vi "SL TAGS Return Unit of Measure Abbreviation.vi"(4 "Unit of Measure":T1=enum."Hour") -> (1 "Seeq Unit of Measure Abbreviation":string)   [LabVIEW 2017, in "EEISysLink.lvclass"]
doc: "Convert selected units to Seeq supported unit abbreviation string\n\nJames Tillett\nEndeavor Engineering Inc.\nwww.endeavoreng.com"
uses:
  EEISysLink.lvclass
  Controls/SL Tag Unit of Measure.ctl
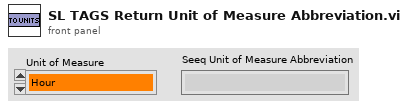
[diagram p1: front panel]
types:
  T1 = typedef "EEISysLink.lvclass/SL Tag Unit of Measure.ctl" = enum16{"no units", "Second", "Hour", "Minute", "Day", "Year", "Month", "Week", "Foot", "Yard", "Meter", "Centimeter", "Inch", "Mile", "Nautical Mile", "Miles per Hour", "Meters per second", "Square meter", "Cubic meter", "Cubic centimeter", "Cubic inch", "Liter", "Gallon", "Gallons dry US", "Gallon UK", "Percent", "Revolutions per minute", "Revolution", "Degree angle", "Astronomical Unit", "Atom", "Atomic mass", "Bar", "Byte", "C (speed of light)", "Curie", "Decibel", "Electron Volt", "Ounce", "Knot", "G", "Grade", "Are", "Hectare", "Faraday", "Franklin", "Gilbert", "Erg", "Lambert", "Maxwell", "Gauss", "Electron mass", "Kilogram force", "Pound force", "Rad", "Centiradian", "Sphere", "Mach", "Fluid Ounces", "Fluid Ounces UK", "Fahrenheit", "Celsius", "Kelvin", "Rankine", "Gram", "Kilogram", "Pound", "Short/US Ton", "Long/UK ton", "Metric ton", "Mole", "Pounds per square inch", "Inches water column", "Torr", "Millitorr", "Millimeter mercury", "Inches mercury", "Bar (2)", "Atmosphere", "Pascal", "Watt", "kiloWatt", "Horsepower", "Kilowatt Hour", "British thermal units", "Millions of BTU", "Ampere", "Candela", "Radian", "Steradian", "Bit", "Hertz", "Newton", "Joule", "Coulomb", "Volt", "Farad", "Ohm", "Siemens", "Weber", "Tesla", "Henry", "Lumen", "Lux", "Becqueral", "Gray", "Sievert", "Katal", "Angstrom", "Light Year", "Parsec", "Point", "Pixel", "Dyne", "Kilogram force (2)", "Pound force (2)", "Rem", "Rutherford", "Roentgen"}
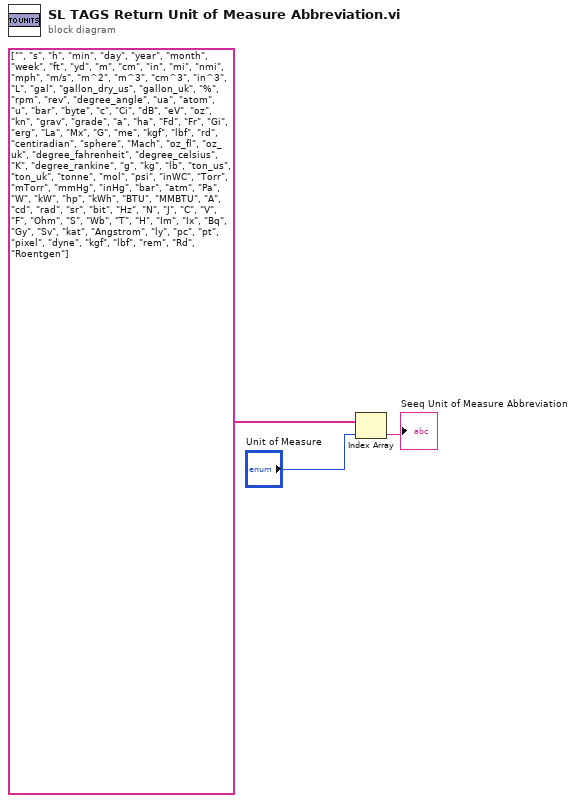
[diagram p0: block diagram]
diagram:
  n1 = Index Array(array=string[] ["", "s", "h", "min", "day", "year", "month", "week", "ft", "yd", "m", "cm", "in", "mi", "nmi", "mph", "m/s", "m^2", "m^3", "cm^3", "in^3", "L", "gal", "gallon_dry_us", "gallon_uk", "%", "rpm", "rev", "degree_angle", "ua", "atom", "u", "bar", "byte", "c", "Ci", "dB", "eV", "oz", "kn", "grav", "grade", "a", "ha", "Fd", "Fr", "Gi", "erg", "La", "Mx", "G", "me", "kgf", "lbf", "rd", "centiradian", "sphere", "Mach", "oz_fl", "oz_uk", "degree_fahrenheit", "degree_celsius", "K", "degree_rankine", "g", "kg", "lb", "ton_us", "ton_uk", "tonne", "mol", "psi", "inWC", "Torr", "mTorr", "mmHg", "inHg", "bar", "atm", "Pa", "W", "kW", "hp", "kWh", "BTU", "MMBTU", "A", "cd", "rad", "sr", "bit", "Hz", "N", "J", "C", "V", "F", "Ohm", "S", "Wb", "T", "H", "Im", "Ix", "Bq", "Gy", "Sv", "kat", "Angstrom", "ly", "pc", "pt", "pixel", "dyne", "kgf", "lbf", "rem", "Rd", "Roentgen"], index="Unit of Measure") -> (element=→"Seeq Unit of Measure Abbreviation":string)
